vi "Launch Series.vi"(6 "Series CFG":string, 8 "error in":errorcluster, 9 "Virt Instrs":string, 10 "Instr CFGs":string[](array[string]), 11 "Study Actor in":refnum<class "Study Actor.lvclass">) -> (0 "error out":errorcluster, 3 "Study Actor out":refnum<class "Study Actor.lvclass">)   [LabVIEW 2023, in "Study Actor.lvlib" / "Study Actor.lvclass"]
uses:
  Study Actor.lvclass
  C:/Program Files/National Instruments/LabVIEW 2023/vi.lib/MGI/Panel Manager/Panel Actor/Panel Actor/Panel Actor.lvclass
  Series/Series Actor/Series Actor/Series Actor.lvclass
  Study Actor.lvclass/Study Actor.ctl
  Series/Series Actor/Series Actor/Series Actor.lvclass/Series Actor.ctl
  HAL/MSS Target Actor/IMSS Target Actor Messages/Init Instruments Msg/Init Instruments Msg.lvclass/Init Instruments Msg.ctl
  <vilib>/ActorFramework/Message Enqueuer/Message Enqueuer.lvclass/Message Enqueuer.ctl
  HAL/MSS Target Actor/IMSS Target Actor Messages/Init Virtual Instruments Msg/Init Virtual Instruments Msg.lvclass/Init Virtual Instruments Msg.ctl
  6bf2b5dd-dbe1-4461-bebd-9ea40a2179ed.vi
  6bf2b5dd-dbe1-4461-bebd-9ea40a2179ed.vi/a4169a97-72fc-4003-a778-603cf20cafa0.vi
  <vilib>/ActorFramework/Message Enqueuer/Enqueue.vi
  <vilib>/JDP Science/JSONtext/Find Item.vi
  <vilib>/JDP Science/JSONtext/Next JSON Value.vi
  <vilib>/JDP Science/JSONtext/String Subset.vi
  <vilib>/JDP Science/JSONtext/Parsing/Advance past next JSON Value (inlined COPY).vi
  <vilib>/JDP Science/JSONtext/Parsing/Advance past whitespace.vi
  <vilib>/JDP Science/JSONtext/Parsing/Advance past String.vi
  <vilib>/JDP Science/JSONtext/Parsing/Advance past Number.vi
  <vilib>/JDP Science/JSONtext/Parsing/Advance past Line Ending.vi
  HAL/MSS Target Actor/IMSS Target Actor Messages/Init Instruments Msg/Init Instruments Msg.lvclass
  C:/Program Files/National Instruments/LabVIEW 2023/vi.lib/ActorFramework/Message/Message.lvclass
  HAL/MSS Target Actor/IMSS Target Actor Messages/Init Virtual Instruments Msg/Init Virtual Instruments Msg.lvclass
  <vilib>/MGI/Panel Manager/Panel/Panel/Subpanel/Subpanel.lvclass
  C:/Program Files/National Instruments/LabVIEW 2023/vi.lib/MGI/Panel Manager/Panel/Panel/Panel.lvclass
  <vilib>/JDP Science/JSONtext/Parsing/Parse Full Path or Item Name.vi
  <vilib>/JDP Science/JSONtext/Parsing/Advance past Array.vi
  <vilib>/JDP Science/JSONtext/Parsing/Advance past Object.vi
  <vilib>/JDP Science/JSONtext/support/Error Cluster From Code.vi
  <vilib>/JDP Science/JSONtext/Offset/Find Item Locations by Path.vi
  <vilib>/JDP Science/JSONtext/JSON text to Variant.vi
  <vilib>/Utility/error.llb/Error Cluster From Error Code.vi
  <vilib>/Utility/LVClass/Get LV Class Name.vi
  <resource>/AFDebug/Generate Trace for Message.vi
  <vilib>/ActorFramework/Message Priority Queue/Priority Enqueue.vi
  <vilib>/MGI/Panel Manager/Panel/Panel/Subpanel/Subpanel.vi
  <vilib>/JDP Science/JSONtext/LVClass Serializer/JSONtext LVClass Serializer.lvclass
  <vilib>/MGI/Panel Manager/Panel Actor/Panel Actor/Panel Actor.lvclass
  <vilib>/MGI/Panel Manager/Panel/Panel.lvlib
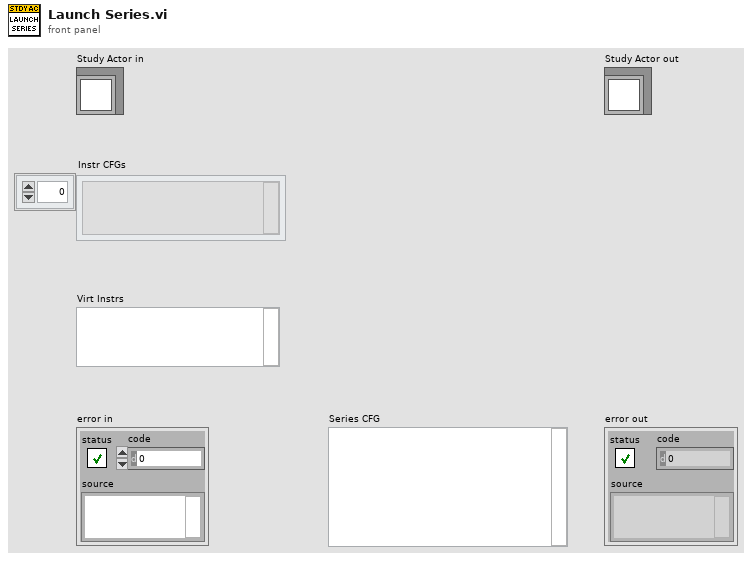
[diagram p1: front panel]
types:
  T1 = cluster{"Task-Point Ident":string, "Instr Ident":string, "Const Action Data":string, "Class":string}[]
  T2 = map{string, refnum<class "Message Enqueuer.lvclass">}
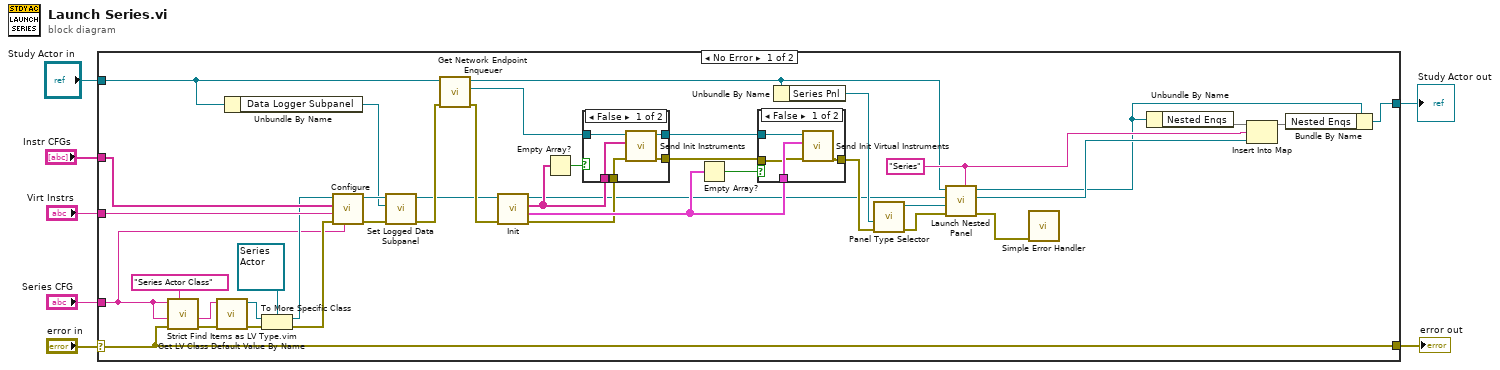
[diagram p0: block diagram]
diagram:
  n1 = case shown="No Error" "error in" {
    selector: "error in" -> [w11 w60]
    tunnel: [w11 w60] -> w6
    tunnel: [w33 w59] -> w4
    tunnel: "Study Actor in" -> [w9 w59]
    tunnel: "Series CFG" -> [w12 _]
    tunnel: "Instr CFGs" -> [w40 _]
    tunnel: "Virt Instrs" -> [w39 _]
    frame No Error {
      w37 = "Series" ("Debug Alias")
      n2 = call "Strict Find Items as LV Type.vim"("$Path or Item Name"="Series Actor Class", "error in"=w11, "Data Type and Default Value"=w12, "<JSON>"=w12) -> ("error out"=w41:errorcluster, "Data out"=w42:string)  [unwired: 5 in, 1 out]
      n3 = call <vilib>:"Get LV Class Default Value By Name.vi"("error in (no error)"=w41, "class name"=w42) -> ("error out"=w45:errorcluster, "object"=w44:refnum<class>)  [unwired: 8 in]
      n4 = Unbundle By Name(w9) -> ("Data Logger Subpanel"=w8:refnum<vi>)
      n5 = To More Specific Class(target class=refnum<class "Series Actor.lvclass"> refnum ("Series Actor.lvlib:Series Actor.lvclass"), reference=w44, error in=w45) -> (specific class reference=w16:refnum<class "Series Actor.lvclass">, error out=w17:errorcluster)
      n6 = call "Configure.vi"("Series CFG"=w12, "error in"=w17, "Virt Instrs"=w39, "Instr CFGs"=w40, "Series Actor in"=w16) -> ("error out"=w28:errorcluster, "Series Actor out"=w46:refnum<class "Series Actor.lvclass">)  [unwired: 5 in]
      n7 = call "Set Logged Data Subpanel.vi"("Data Logger Subpanel"=w8, "Series Actor in"=w46) -> ("Series Actor out"=w10:refnum<class "Series Actor.lvclass">)  [unwired: 9 in]
      n8 = call "Get Network Endpoint Enqueuer.vi"("error in"=w28, "Study Actor in"=w9) -> ("error out"=w27:errorcluster, "Network Endpoint Enqueuer"=w26:refnum<class "Message Enqueuer.lvclass">, "Study Actor out"=w18:refnum<class "Study Actor.lvclass">)  [unwired: 6 in, 1 out]
      n9 = call "Init.vi"("error in"=w27, "Series Actor in"=w10) -> ("error out"=w20:errorcluster, "Target Virt Instrs"=w21:T1, "Target Physical Instr CFGs"=w25:string[], "Series Actor out"=w13:refnum<class "Series Actor.lvclass">)  [unwired: 6 in]
      n10 = Empty Array?(array=w25) -> (empty?=w23:bool)
      n11 = case shown="False" w23 {
        tunnel: w26 -> [w51 w52]
        tunnel: w25 -> [w50 _]
        tunnel: [w49 w52] -> w24
        tunnel: w20 -> [w48 w53]
        tunnel: [w47 w53] -> w19
        frame False {
          n12 = call "Send Init Instruments.vi"("error in (no error)"=w48, "Physical Instr CFGs"=w50, "Message Enqueuer"=w51) -> ("error out"=w47:errorcluster, "Message Enqueuer out"=w49:refnum<class "Message Enqueuer.lvclass">)  [unwired: 7 in]
        }
        frame True {
        }
      }
      n13 = Empty Array?(array=w21) -> (empty?=w22:bool)
      n14 = case shown="False" w22 {
        tunnel: w21 -> [w57 _]
        tunnel: w24 -> [w56 _]
        tunnel: w19 -> [w55 w58]
        tunnel: [w54 w58] -> w14
        frame False {
          n15 = call "Send Init Virtual Instruments.vi"("error in (no error)"=w55, "Virt Instrs"=w57, "Message Enqueuer"=w56) -> ("error out"=w54:errorcluster)  [unwired: 7 in, 1 out]
        }
        frame True {
        }
      }
      n16 = Unbundle By Name(w18) -> ("Series Pnl"=w30:refnum<vi>)
      n17 = call-poly <vilib>:"Panel Type Selector.vi"("Error In"=w14, "Sub Panel"=w30) -> ("Error Out"=w31:errorcluster, "Subpanel Out"=w29:refnum<class "Subpanel.lvclass">)  [unwired: 8 in]
      n18 = call <vilib>:"Launch Nested Panel.vi"("Debug Alias"=w37, "error in (no error)"=w31, "Panel"=w29, "Nested Panel Actor"=w13, "Panel Actor in"=w18) -> ("error out"=w35:errorcluster, "Nested Actor's Enqueuer"=w36:refnum<class "Message Enqueuer.lvclass">, "Panel Actor out"=w34:refnum<class "Study Actor.lvclass">)  [unwired: 3 in, 1 out]
      n19 = call <vilib>:"Simple Error Handler.vi"("error in (no error)"=w35) -> ()  [unwired: 4 in, 5 out]
      n20 = Unbundle By Name(w34) -> ("Nested Enqs"=w38:T2)
      n21 = Insert Into Map(map in=w38, key=w37, value=w36) -> (map out=w32:T2)  [unwired: 2 out]
      n22 = Bundle By Name(cluster=w34, "Nested Enqs"=w32) -> (w33:refnum<class "Study Actor.lvclass">)
    }
    frame Error {
    }
  }
  "error out" <- w6
  "Study Actor out" <- w4
